vi "writeToXML.vi"(8 "error in (no error)":errorcluster, 10 "ClassLabel":string, 11 "TCSIersCommand in":refnum<class "TCSIersCommand.lvclass">) -> (0 "error out":errorcluster, 2 "XMLout":string, 3 "TCSIersCommand out":refnum<class "TCSIersCommand.lvclass">)   [LabVIEW 2014, in "TCSDataDefinitions.lvlib" / "TCSTimeComponentCommand.lvlib" / "TCSIersCommand.lvclass"]
uses:
  TCSIersCommand.lvclass
  TCSCommand/TCSCommand/TCSCommand.lvclass
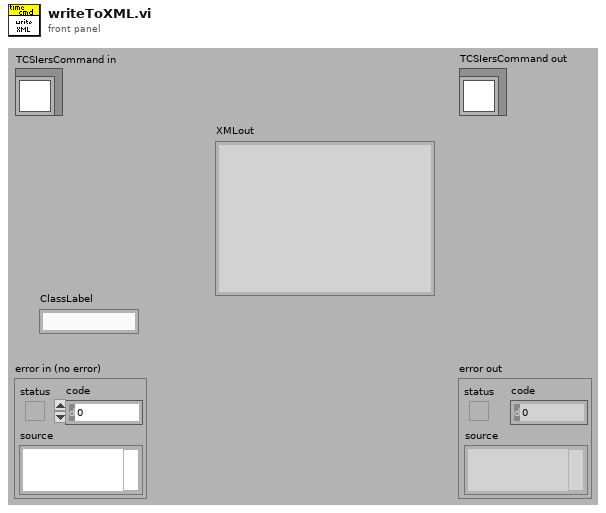
[diagram p1: front panel]
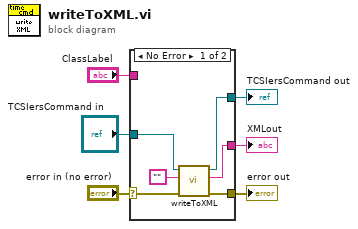
[diagram p0: block diagram]
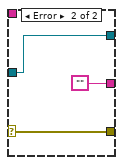
[diagram p2: hidden frame]
diagram:
  n1 = case shown="No Error" "error in (no error)" {
    selector: "error in (no error)" -> [w11 w15]
    tunnel: [w10 w15] -> w5
    tunnel: [w7 w14] -> w4
    tunnel: "TCSIersCommand in" -> [w8 w14]
    tunnel: [w9 ""] -> w3
    tunnel: "ClassLabel" -> [_ _]
    frame No Error {
      n2 = call-parent "writeToXML.vi"("error in (no error)"=w11, "Class Label"="", "TCSCommand in"=w8) -> ("error out"=w10:errorcluster, "XML out"=w9:string, "TCSCommand out"=w7:refnum<class "TCSIersCommand.lvclass">)  [unwired: 6 in]
    }
    frame Error {
    }
  }
  "error out" <- w5
  "TCSIersCommand out" <- w4
  "XMLout" <- w3
